vi "API TESTERS BUTTONS.vi"() -> ()   [LabVIEW 2024]
doc: "This VI can be used as a launcher VI for the main application or as a debugging tool.\n_____\nBased on DQMH Dev Tools: Project Template 7.1.0.1503."
panel:
  in  "Launch Settings Editor API Tester":bool
  in  "Launch Logger API Tester":bool
  in  "Launch Acquisition API Tester":bool
  in  "Launch CML UI API Tester":bool
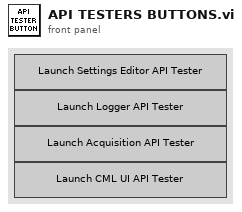
[diagram p1: front panel]
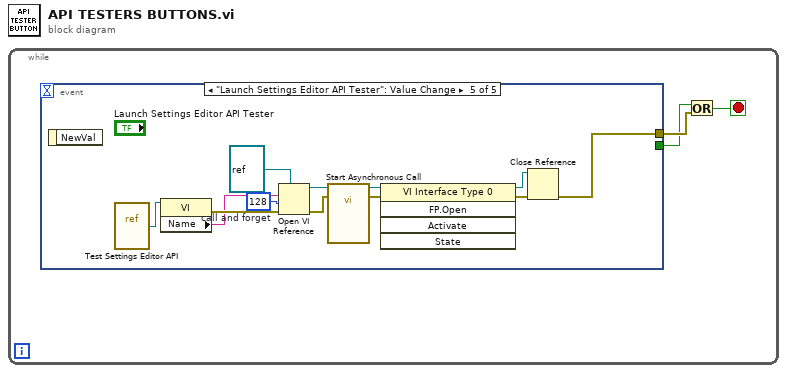
[diagram p0: block diagram]
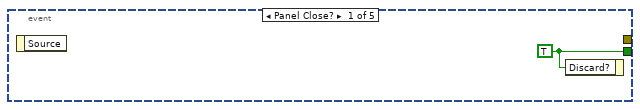
[diagram p2: hidden frame]
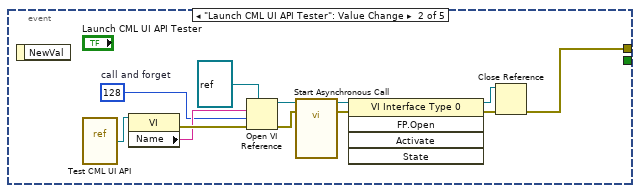
[diagram p3: hidden frame]
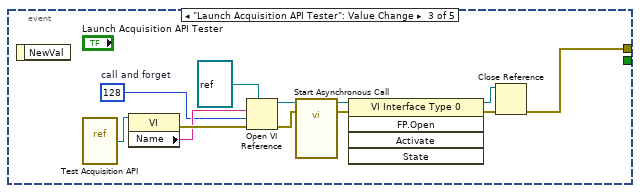
[diagram p4: hidden frame]
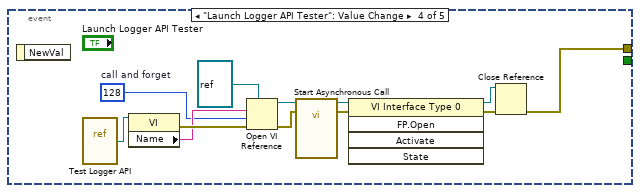
[diagram p5: hidden frame]
diagram:
  n1 = while {
    stop <- w1 stop-if-true
    n2 = event shown="[4] \"Launch Settings Editor API Tester\": Value Change" {
      selector: _ -> [_ _ _ _ _]
      dyn-events: _ -> [_ _ _ _ _]
      timeout: _ -> [_ _ _ _ _]
      tunnel: [w4 _ _ _ _] -> w2
      tunnel: [_ w12 w24 w36 w48] -> w3
      event Panel Close? {
        w4 = TRUE ("Discard?")
        n3 = event-data() -> ()  [unwired: 1 in, 1 out]
        n4 = event-data ("Event Filter Node")("Discard?"=w4) -> ()  [unwired: 1 in, 1 out]
      }
      event "Launch CML UI API Tester": Value Change {
        w5 = 128  # call and forget
        n5 = event-data() -> ()  [unwired: 1 in, 1 out]
        n6 = vi-ref "Test CML UI API.vi"() -> (w11:refnum<vi>)
        n7 = property class="VI"(reference=w11) -> (error out=w16:errorcluster, "Name"=w10:string)  [unwired: 1 in, 1 out]
        n8 = Open VI Reference(type specifier VI Refnum (for type only)=refnum<vi> refnum, vi path=w10, options=w5, error in (no error)=w16) -> (vi reference=w8:refnum<vi>, error out=w15:errorcluster)  [unwired: 2 in]
        n9 = call-by-ref "Start Asynchronous Call"(reference=w8, error in=w15) -> (reference out=w7:refnum<vi>, error out=w14:errorcluster)  [unwired: 12 in]
        n10 = invoke class="VI Interface Type 0" method="FP.Open"(reference=w7, error in=w14) -> (reference out=w6:refnum<vi>, error out=w13:errorcluster)  [unwired: 3 in, 3 out]
        n11 = Close Reference(reference=w6, error in (no error)=w13) -> (error out=w12:errorcluster)
      }
      event "Launch Acquisition API Tester": Value Change {
        w17 = 128  # call and forget
        n12 = event-data() -> ()  [unwired: 1 in, 1 out]
        n13 = vi-ref "Test Acquisition API.vi"() -> (w23:refnum<vi>)
        n14 = property class="VI"(reference=w23) -> (error out=w28:errorcluster, "Name"=w22:string)  [unwired: 1 in, 1 out]
        n15 = Open VI Reference(type specifier VI Refnum (for type only)=refnum<vi> refnum, vi path=w22, options=w17, error in (no error)=w28) -> (vi reference=w20:refnum<vi>, error out=w27:errorcluster)  [unwired: 2 in]
        n16 = call-by-ref "Start Asynchronous Call"(reference=w20, error in=w27) -> (reference out=w19:refnum<vi>, error out=w26:errorcluster)  [unwired: 12 in]
        n17 = invoke class="VI Interface Type 0" method="FP.Open"(reference=w19, error in=w26) -> (reference out=w18:refnum<vi>, error out=w25:errorcluster)  [unwired: 3 in, 3 out]
        n18 = Close Reference(reference=w18, error in (no error)=w25) -> (error out=w24:errorcluster)
      }
      event "Launch Logger API Tester": Value Change {
        w29 = 128  # call and forget
        n19 = event-data() -> ()  [unwired: 1 in, 1 out]
        n20 = vi-ref "Test Logger API.vi"() -> (w35:refnum<vi>)
        n21 = property class="VI"(reference=w35) -> (error out=w40:errorcluster, "Name"=w34:string)  [unwired: 1 in, 1 out]
        n22 = Open VI Reference(type specifier VI Refnum (for type only)=refnum<vi> refnum, vi path=w34, options=w29, error in (no error)=w40) -> (vi reference=w32:refnum<vi>, error out=w39:errorcluster)  [unwired: 2 in]
        n23 = call-by-ref "Start Asynchronous Call"(reference=w32, error in=w39) -> (reference out=w31:refnum<vi>, error out=w38:errorcluster)  [unwired: 12 in]
        n24 = invoke class="VI Interface Type 0" method="FP.Open"(reference=w31, error in=w38) -> (reference out=w30:refnum<vi>, error out=w37:errorcluster)  [unwired: 3 in, 3 out]
        n25 = Close Reference(reference=w30, error in (no error)=w37) -> (error out=w36:errorcluster)
      }
      event "Launch Settings Editor API Tester": Value Change {
        w41 = 128  # call and forget
        n26 = event-data() -> ()  [unwired: 1 in, 1 out]
        n27 = vi-ref "Test Settings Editor API.vi"() -> (w47:refnum<vi>)
        n28 = property class="VI"(reference=w47) -> (error out=w52:errorcluster, "Name"=w46:string)  [unwired: 1 in, 1 out]
        n29 = Open VI Reference(type specifier VI Refnum (for type only)=refnum<vi> refnum, vi path=w46, options=w41, error in (no error)=w52) -> (vi reference=w44:refnum<vi>, error out=w51:errorcluster)  [unwired: 2 in]
        n30 = call-by-ref "Start Asynchronous Call"(reference=w44, error in=w51) -> (reference out=w43:refnum<vi>, error out=w50:errorcluster)  [unwired: 12 in]
        n31 = invoke class="VI Interface Type 0" method="FP.Open"(reference=w43, error in=w50) -> (reference out=w42:refnum<vi>, error out=w49:errorcluster)  [unwired: 3 in, 3 out]
        n32 = Close Reference(reference=w42, error in (no error)=w49) -> (error out=w48:errorcluster)
      }
    }
    n33 = Or(x=w2, y=w3) -> (x .or. y?=w1:bool)
  }
